vi "terminate.vi"(8 "error in (no error)":errorcluster, 11 "GenericPlugin in":refnum<class "StimulatorDL090503.lvclass">) -> (0 "error out":errorcluster, 3 "GenericPlugin out":refnum<class "StimulatorDL090503.lvclass">)   [LabVIEW 2010, in "StimulatorDL090503.lvclass"]
doc: "The dynamic dispatch version of this VI terminates the plug-in object by releasing all of its resources."
uses:
  StimulatorDL090503.lvclass
  StimulatorDL090503.lvclass/StimulatorDL090503.ctl
  SignalWriter/GenericSignalWriter/GenericSignalWriter/GenericSignalWriter.lvclass
  StimulatorDL090503Scaffold/StimulatorDL090503Scaffold/StimulatorDL090503Scaffold.lvclass
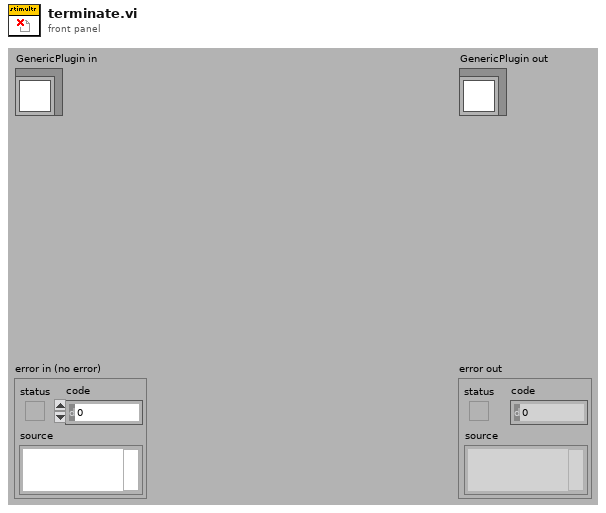
[diagram p1: front panel]
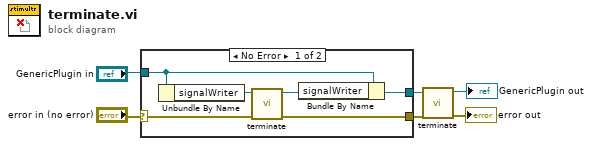
[diagram p0: block diagram]
diagram:
  n1 = case shown="No Error" "error in (no error)" {
    selector: "error in (no error)" -> [w12 w13]
    tunnel: [w11 w13] -> w4
    tunnel: "GenericPlugin in" -> [w9 w14]
    tunnel: [w7 w14] -> w3
    frame No Error {
      n2 = Unbundle By Name(w9) -> ("signalWriter"=w10:refnum<class "GenericSignalWriter.lvclass">)
      n3 = call-dynamic "terminate.vi"("error in (no error)"=w12, "GenericPlugin in"=w10) -> ("error out"=w11:errorcluster, "GenericPlugin out"=w8:refnum<class "GenericSignalWriter.lvclass">)  [unwired: 8 out]
      n4 = Bundle By Name(cluster=w9, "signalWriter"=w8) -> (w7:refnum<class "StimulatorDL090503.lvclass">)
    }
    frame Error {
    }
  }
  n5 = call-parent "terminate.vi"("error in (no error)"=w4, "GenericPlugin in"=w3) -> ("error out"=→"error out":errorcluster, "GenericPlugin out"=→"GenericPlugin out":refnum<class "StimulatorDL090503.lvclass">)  [unwired: 8 in]
